vi "Is valid VI filename.vi"(1 "VI Filename":string) -> (0 "Is VI filename valid?":bool)   [LabVIEW 2022 SP3]
doc: "This VI returns True if and only if the input string is a valid VI filename.\n\nA string is a valid VI filename if:\n1. It contains at least four characters: three for the file extension, and at least one for the file name\n2. It ends in \".vi\" (case-insensitive)"
panel:
  # "Development\nControls or indicators that are useful for development or testing, but which are not outputs of the VI."
  # "Input\nInputs to the VI"
  # "Output\nOutputs of the VI"
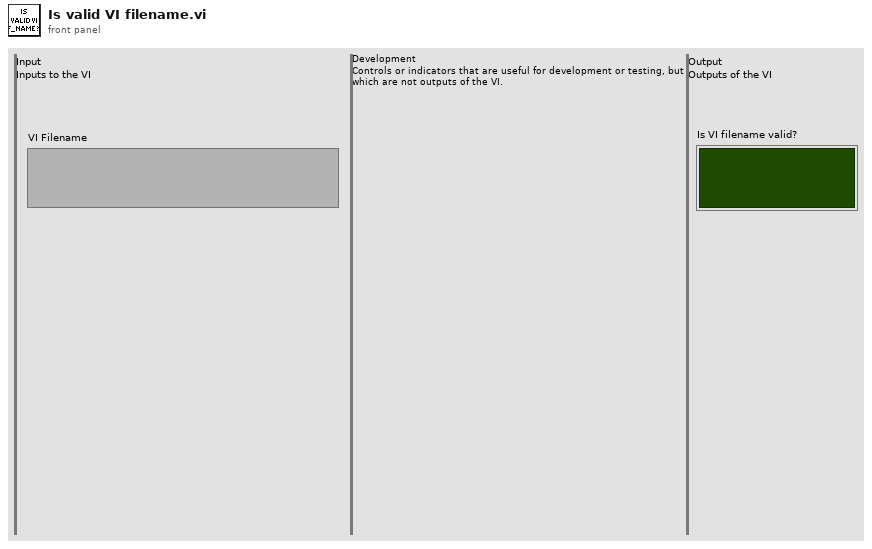
[diagram p1: front panel]
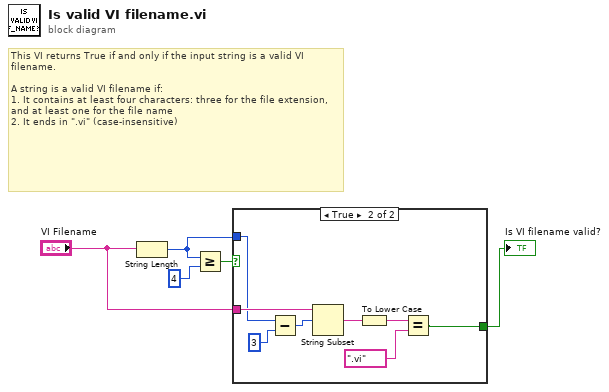
[diagram p0: block diagram]
diagram:
  # "This VI returns True if and only if the input string is a valid VI filename.\n\nA string is a valid VI filename if:\n1. It contains at least four characters: three for the file extension, and at least one for the file name\n2. It ends in \".vi\" (case-insensitive)"
  n1 = String Length(string="VI Filename") -> (length=w2:i32)
  n2 = Greater Or Equal?(x=w2, y=4) -> (x >= y?=w4:bool)
  n3 = case shown="True" w4 {
    tunnel: "VI Filename" -> [_ w13]
    tunnel: w2 -> [_ w11]
    tunnel: [_ w6] -> w1
    frame False {
    }
    frame True {
      n4 = Subtract(x=w11, y=3) -> (x-y=w12:i32)
      n5 = String Subset(string=w13, offset (0)=w12) -> (substring=w9:string)  [unwired: 1 in]
      n6 = To Lower Case(string=w9) -> (all lower case string=w8:string)
      n7 = Equal?(x=w8, y=".vi") -> (x = y?=w6:bool)
    }
  }
  "Is VI filename valid?" <- w1
